vi "BT_pass_fail.vi"(8 "error in":errorcluster, 9 "BT Item result Input":dbl, 10 "BT Item Name Input":string="ACP_MAX_POWER_DBM_OFFSET_-5:", 11 "BT Test Text Input":string="TX_BDR 2402 DH1") -> (0 "error out":errorcluster, 2 "Pass?(string)":string, 3 "Pass?(boolen)":bool)   [LabVIEW 2012]
uses:
  <vilib>/Utility/file.llb/Read From Spreadsheet File (string).vi
panel:
  out "High limit":dbl
  out "Lower limit":dbl
  out "BT_RX_EDR":string[][](array[string])
  out "output 3":string
  out "Frequency":dbl
  out "BT test item":string
  in  "BT_Range":T1={"BT_TX_BDR"=[["POWER_AVERAGE_DBM", "-6", "4", "", "", "", "", "", "", "", "", "", "", "", ""], ["POWER_PEAK_DBM", "", "23", "", "", "", "", "", "", "", "", "", "", "", ""], ["DELTA_F2_MAX_ACCESS", "115", "", "", "", "", "", "", "", "", "", "", "", "", ""], ["ACP_MAX_POWER_DBM_OFFSET_-5", "", "-40", "", "", "", "", "", "", "", "", "", "", "", ""], ["ACP_MAX_POWER_DBM_OFFSET_-4", "", "-40", "", "", "", "", "", "", "", "", "", "", "", ""], ["ACP_MAX_POWER_DBM_OFFSET_-3", "", "-40", "", "", "", "", "", "", "", "", "", "", "", ""], ["ACP_MAX_POWER_DBM_OFFSET_-2", "", "-40", "", "", "", "", "", "", "", "", "", "", "", ""], ["ACP_MAX_POWER_DBM_OFFSET_-1", "", "-20", "", "", "", "", "", "", "", "", "", "", "", ""], ["ACP_MAX_POWER_DBM_OFFSET_1", "", "-20", "", "", "", "", "", "", "", "", "", "", "", ""], ["ACP_MAX_POWER_DBM_OFFSET_2", "", "-40", "", "", "", "", "", "", "", "", "", "", "", ""], ["ACP_MAX_POWER_DBM_OFFSET_3", "", "-40", "", "", "", "", "", "", "", "", "", "", "", ""], ["ACP_MAX_POWER_DBM_OFFSET_4", "", "-40", "", "", "", "", "", "", "", "", "", "", "", ""], ["ACP_MAX_POWER_DBM_OFFSET_5", "", "-40", "", "", "", "", "", "", "", "", "", "", "", ""]], "BT_TX_EDR"=[["EDR_OMEGA_I", "-75", "75", "", "", "", "", "", "", "", "", "", "", "", ""], ["EDR_POW_DIFF_DB", "-4", "1", "", "", "", "", "", "", "", "", "", "", "", ""], ["EDR_EVM_AV", "", "13", "", "", "", "", "", "", "", "", "", "", "", ""], ["EDR_EVM_PK", "", "25", "", "", "", "", "", "", "", "", "", "", "", ""], ["EDR_PROB_EVM_99_PASS", "100", "100", "", "", "", "", "", "", "", "", "", "", "", ""], ["POWER_AVERAGE_DBM", "-6", "4", "", "", "", "", "", "", "", "", "", "", "", ""], ["ACP_MAX_POWER_DBM_OFFSET_-5", "", "-40", "", "", "", "", "", "", "", "", "", "", "", ""], ["ACP_MAX_POWER_DBM_OFFSET_-4", "", "-40", "", "", "", "", "", "", "", "", "", "", "", ""], ["ACP_MAX_POWER_DBM_OFFSET_-3", "", "-40", "", "", "", "", "", "", "", "", "", "", "", ""], ["ACP_MAX_POWER_DBM_OFFSET_-2", "", "-20", "", "", "", "", "", "", "", "", "", "", "", ""], ["ACP_MAX_POWER_DB_OFFSET_-1", "", "-26", "", "", "", "", "", "", "", "", "", "", "", ""], ["ACP_MAX_POWER_DB_OFFSET_1", "", "-26", "", "", "", "", "", "", "", "", "", "", "", ""], ["ACP_MAX_POWER_DBM_OFFSET_2", "", "-20", "", "", "", "", "", "", "", "", "", "", "", ""], ["ACP_MAX_POWER_DBM_OFFSET_3", "", "-40", "", "", "", "", "", "", "", "", "", "", "", ""], ["ACP_MAX_POWER_DBM_OFFSET_4", "", "-40", "", "", "", "", "", "", "", "", "", "", "", ""], ["ACP_MAX_POWER_DBM_OFFSET_5", "", "-40", "", "", "", "", "", "", "", "", "", "", "", ""]], "BT_RX_BDR"=[["BER", "", "0.1", "", "", "", "", "", "", "", "", "", "", "", ""]], "BT_RX_EDR"=[["BER", "", "0.1", "", "", "", "", "", "", "", "", "", "", "", ""]]}
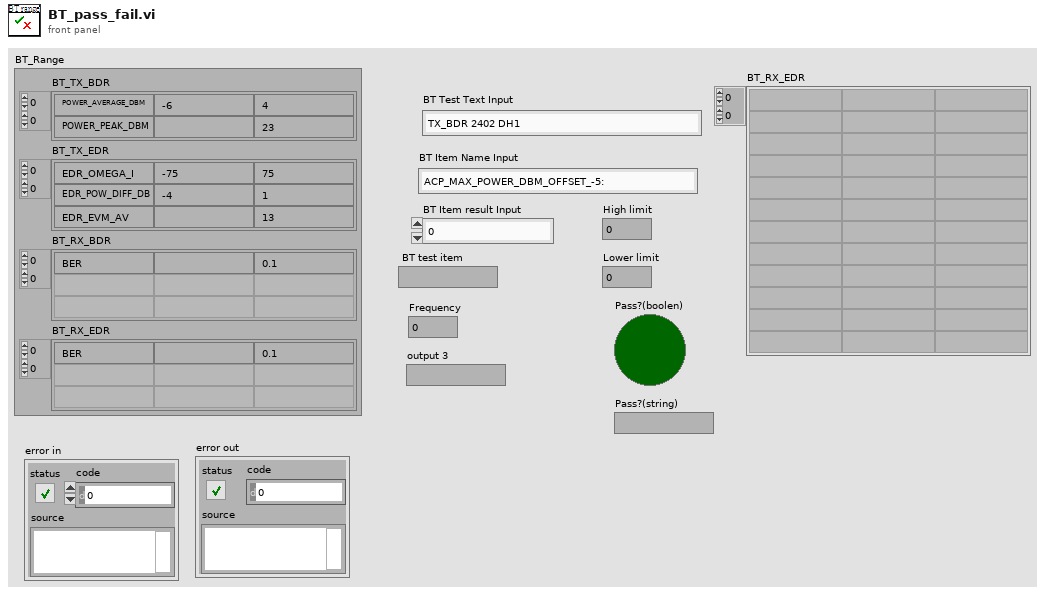
[diagram p1: front panel]
types:
  T1 = cluster{"BT_TX_BDR":string[][], "BT_TX_EDR":string[][], "BT_RX_BDR":string[][], "BT_RX_EDR":string[][]}
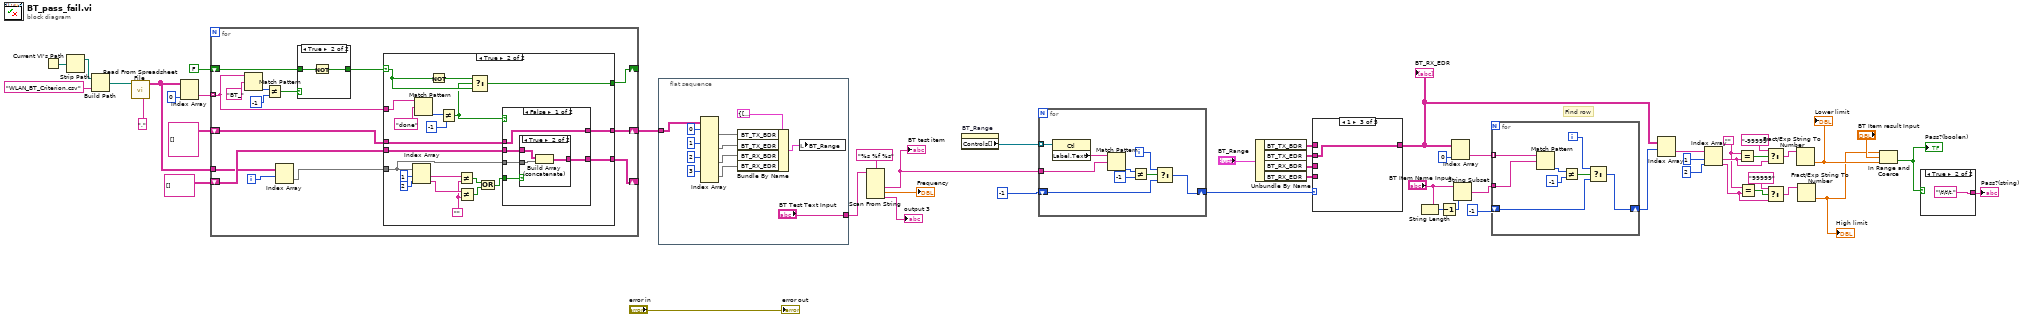
[diagram p0: block diagram]
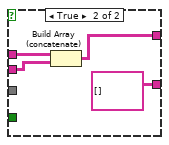
[diagram p4: hidden frame]
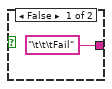
[diagram p6: hidden frame]
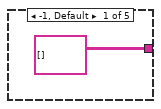
[diagram p7: hidden frame]
diagram:
  w23 = ""
  # "Find row"
  n1 = Current VI's Path() -> (path=w13:path)
  n2 = Strip Path(path=w13) -> (stripped path=w12:path)  [unwired: 1 out]
  n3 = Build Path(base path=w12, name or relative path="WLAN_BT_Criterion.csv") -> (appended path=w10:path)
  n4 = call-poly <vilib>:"Read From Spreadsheet File.vi"("delimiter (\\t)"="," ("delimiter (\\t)"), "file path (dialog if empty)"=w10) -> ("all rows"=w4:string[][])  [unwired: 5 in, 4 out]
  n5 = Index Array(array=w4, index (col)=0 ("disabled index (col)")) -> (element=w5:string[])  [unwired: 1 in]
  n6 = for {
    tunnel: w5 -> [w56] mode=indexing
    shift-right: [w55] -> _
    shift-left: FALSE ("Strat to store date") -> [w63]
    shift-right: [w60] -> _
    shift-left: string[][] [] -> [w61]
    tunnel: w4 -> [w59]
    shift-right: [w53] -> w1
    shift-left: string[][][] [] -> [w54]
    i -> [w58]
    n7 = Match Pattern(string=w56, regular expression="BT_") -> (offset past match=w66:i32)  [unwired: 1 in, 3 out]
    n8 = Not Equal?(x=w66, y=-1) -> (x != y?=w64:bool)
    n9 = Index Array(array=w59, index (row)=w58) -> (element=w57:string[])  [unwired: 1 in]
    n10 = case shown="True" w64 {
      tunnel: [w105 w106] -> w62
      tunnel: w63 -> [w105 w107]
      frame False {
      }
      frame True {
        n11 = Not(x=w107) -> (.not. x?=w106:bool)
      }
    }
    n12 = case shown="True" w62 {
      selector: w62 -> [w69 w78]
      tunnel: w61 -> [w70 w84]
      tunnel: w57 -> [_ w74]
      tunnel: [w70 w83] -> w60
      tunnel: w56 -> [_ w81]
      tunnel: [w69 w76] -> w55
      tunnel: w54 -> [w68 w72]
      tunnel: [w68 w71] -> w53
      frame False {
      }
      frame True {
        w87 = ""
        n13 = Index Array(array=w74, index #1=1 ("index"), index #2=2 ("index")) -> (element #1=w89:string, element #2=w88:string)
        n14 = Match Pattern(string=w81, regular expression="done") -> (offset past match=w80:i32)  [unwired: 1 in, 3 out]
        n15 = Not(x=w78) -> (.not. x?=w77:bool)
        n16 = Not Equal?(x=w80, y=-1) -> (x != y?=w73:bool)
        n17 = Not Equal?(x=w89, y=w87) -> (x != y?=w86:bool)
        n18 = Not Equal?(x=w88, y=w87) -> (x != y?=w85:bool)
        n19 = Select(t=w77, s=w73, f=w78) -> (s? t:f=w76:bool)
        n20 = Or(x=w86, y=w85) -> (x .or. y?=w75:bool)
        n21 = case shown="False" w73 {
          tunnel: w84 -> [w96 w102]
          tunnel: [w95 string[][] []] -> w83
          tunnel: w75 -> [w94 _]
          tunnel: w74 -> [w93 _]
          tunnel: w72 -> [w92 w103]
          tunnel: [w92 w101] -> w71
          frame False {
            n22 = case shown="True" w94 {
              tunnel: w96 -> [w97 w100]
              tunnel: [w97 w99] -> w95
              tunnel: w93 -> [_ w98]
              frame False {
              }
              frame True {
                n23 = Build Array (concatenate)(w100, w98) -> (w99:string[][])
              }
            }
          }
          frame True {
            n24 = Build Array (concatenate)(w103, w102) -> (w101:string[][][])
          }
        }
      }
    }
  }
  n25 = flat-sequence {
    tunnel: ["BT Test Text Input"] -> w52
    tunnel: w1 -> [w118]
    frame #0 {
      n26 = Index Array(array=w118, index (dim 0) #1=0 ("index (page)"), index (dim 0) #2=1 ("index (page)"), index (dim 0) #3=2 ("index (page)"), index (dim 0) #4=3 ("index (page)")) -> (element #1=w111:string[][], element #2=w110:string[][], element #3=w109:string[][], element #4=w108:string[][])  [unwired: 8 in]
      n27 = Bundle By Name(cluster=T1 {"BT_TX_BDR"=[["POWER_AVERAGE_DBM", "-6", "4", "", "", "", "", "", "", "", "", "", "", "", ""], ["POWER_PEAK_DBM", "", "23", "", "", "", "", "", "", "", "", "", "", "", ""], ["DELTA_F2_MAX_ACCESS", "115", "", "", "", "", "", "", "", "", "", "", "", "", ""], ["ACP_MAX_POWER_DBM_OFFSET_-5", "", "-40", "", "", "", "", "", "", "", "", "", "", "", ""], ["ACP_MAX_POWER_DBM_OFFSET_-4", "", "-40", "", "", "", "", "", "", "", "", "", "", "", ""], ["ACP_MAX_POWER_DBM_OFFSET_-3", "", "-40", "", "", "", "", "", "", "", "", "", "", "", ""], ["ACP_MAX_POWER_DBM_OFFSET_-2", "", "-40", "", "", "", "", "", "", "", "", "", "", "", ""], ["ACP_MAX_POWER_DBM_OFFSET_-1", "", "-20", "", "", "", "", "", "", "", "", "", "", "", ""], ["ACP_MAX_POWER_DBM_OFFSET_1", "", "-20", "", "", "", "", "", "", "", "", "", "", "", ""], ["ACP_MAX_POWER_DBM_OFFSET_2", "", "-40", "", "", "", "", "", "", "", "", "", "", "", ""], ["ACP_MAX_POWER_DBM_OFFSET_3", "", "-40", "", "", "", "", "", "", "", "", "", "", "", ""], ["ACP_MAX_POWER_DBM_OFFSET_4", "", "-40", "", "", "", "", "", "", "", "", "", "", "", ""], ["ACP_MAX_POWER_DBM_OFFSET_5", "", "-40", "", "", "", "", "", "", "", "", "", "", "", ""]], "BT_TX_EDR"=[["EDR_OMEGA_I", "-75", "75", "", "", "", "", "", "", "", "", "", "", "", ""], ["EDR_POW_DIFF_DB", "-4", "1", "", "", "", "", "", "", "", "", "", "", "", ""], ["EDR_EVM_AV", "", "13", "", "", "", "", "", "", "", "", "", "", "", ""], ["EDR_EVM_PK", "", "25", "", "", "", "", "", "", "", "", "", "", "", ""], ["EDR_PROB_EVM_99_PASS", "100", "100", "", "", "", "", "", "", "", "", "", "", "", ""], ["POWER_AVERAGE_DBM", "-6", "4", "", "", "", "", "", "", "", "", "", "", "", ""], ["ACP_MAX_POWER_DBM_OFFSET_-5", "", "-40", "", "", "", "", "", "", "", "", "", "", "", ""], ["ACP_MAX_POWER_DBM_OFFSET_-4", "", "-40", "", "", "", "", "", "", "", "", "", "", "", ""], ["ACP_MAX_POWER_DBM_OFFSET_-3", "", "-40", "", "", "", "", "", "", "", "", "", "", "", ""], ["ACP_MAX_POWER_DBM_OFFSET_-2", "", "-20", "", "", "", "", "", "", "", "", "", "", "", ""], ["ACP_MAX_POWER_DB_OFFSET_-1", "", "-26", "", "", "", "", "", "", "", "", "", "", "", ""], ["ACP_MAX_POWER_DB_OFFSET_1", "", "-26", "", "", "", "", "", "", "", "", "", "", "", ""], ["ACP_MAX_POWER_DBM_OFFSET_2", "", "-20", "", "", "", "", "", "", "", "", "", "", "", ""], ["ACP_MAX_POWER_DBM_OFFSET_3", "", "-40", "", "", "", "", "", "", "", "", "", "", "", ""], ["ACP_MAX_POWER_DBM_OFFSET_4", "", "-40", "", "", "", "", "", "", "", "", "", "", "", ""], ["ACP_MAX_POWER_DBM_OFFSET_5", "", "-40", "", "", "", "", "", "", "", "", "", "", "", ""]], "BT_RX_BDR"=[["BER", "", "0.1", "", "", "", "", "", "", "", "", "", "", "", ""]], "BT_RX_EDR"=[["BER", "", "0.1", "", "", "", "", "", "", "", "", "", "", "", ""]]} ("BT_Range"), "BT_TX_BDR"=w111, "BT_TX_EDR"=w110, "BT_RX_BDR"=w109, "BT_RX_EDR"=w108) -> (w112:T1)
      n28 = local write "BT_Range"(w112) -> ()
    }
  }
  n29 = Scan From String(format string="%s %f %s", input string=w52) -> (output 1=w46:string, output 2=→"Frequency":dbl, output 3=→"output 3":string)  [unwired: 5 in, 3 out]
  "BT test item" <- w46
  n30 = property on="BT_Range" class="Clust (strict)"() -> ("Controls[]"=w48:refnum<vi>[])  [unwired: 2 in, 2 out]
  n31 = for {
    tunnel: w48 -> [w128] mode=indexing
    tunnel: w46 -> [w126]
    shift-right: [w120] -> w44
    shift-left: -1 -> [w121]
    i -> [w122]
    n32 = property class="Ctl"(reference=w128) -> ("Label.Text"=w127:string)  [unwired: 1 in, 2 out]
    n33 = Match Pattern(string=w127, regular expression=w126) -> (offset past match=w125:i32)  [unwired: 1 in, 3 out]
    n34 = Not Equal?(x=w125, y=-1) -> (x != y?=w123:bool)
    n35 = Select(t=w122, s=w123, f=w121) -> (s? t:f=w120:i32)
  }
  n36 = Unbundle By Name("BT_Range") -> ("BT_TX_BDR"=w43:string[][], "BT_TX_EDR"=w42:string[][], "BT_RX_BDR"=w41:string[][], "BT_RX_EDR"=w40:string[][])
  n37 = case shown="1" w44 {
    tunnel: w43 -> [_ w130 _ _ _]
    tunnel: w42 -> [_ _ w131 _ _]
    tunnel: w41 -> [_ _ _ w132 _]
    tunnel: w40 -> [_ _ _ _ w133]
    tunnel: [string[][] [] ("BT_RX_EDR") w130 w131 w132 w133] -> w32
    frame -1, Default {
    }
    frame 0 {
    }
    frame 1 {
    }
    frame 2 {
    }
    frame 3 {
    }
  }
  "BT_RX_EDR" <- w32
  n38 = String Length(string="BT Item Name Input") -> (length=w35:i32)
  n39 = Decrement(x=w35) -> (x-1=w34:i32)
  n40 = Index Array(array=w32, index (col)=0 ("disabled index (col)")) -> (element=w38:string[])  [unwired: 1 in]
  n41 = String Subset(string="BT Item Name Input", length (rest)=w34) -> (substring=w33:string)  [unwired: 1 in]
  n42 = for {
    tunnel: w38 -> [w141] mode=indexing
    tunnel: w33 -> [w140]
    shift-right: [w134] -> w31
    shift-left: -1 -> [w135]
    i -> [w136]
    n43 = Match Pattern(string=w141, regular expression=w140) -> (offset past match=w139:i32)  [unwired: 1 in, 3 out]
    n44 = Not Equal?(x=w139, y=-1) -> (x != y?=w137:bool)
    n45 = Select(t=w136, s=w137, f=w135) -> (s? t:f=w134:i32)
  }
  n46 = Index Array(array=w32, index (row)=w31) -> (element=w30:string[])  [unwired: 1 in]
  n47 = Index Array(array=w30, index #1=1 ("index"), index #2=2 ("index")) -> (element #1=w26:string, element #2=w22:string)
  n48 = Equal?(x=w23, y=w26) -> (x = y?=w27:bool)
  n49 = Equal?(x=w23, y=w22) -> (x = y?=w24:bool)
  n50 = Select(t="-99999", s=w27, f=w26) -> (s? t:f=w20:string)
  n51 = Select(t="99999", s=w24, f=w22) -> (s? t:f=w19:string)
  n52 = Fract/Exp String To Number(string=w20) -> (number=w17:dbl)  [unwired: 3 in, 1 out]
  "Lower limit" <- w17
  n53 = Fract/Exp String To Number(string=w19) -> (number=w16:dbl)  [unwired: 3 in, 1 out]
  "High limit" <- w16
  n54 = In Range and Coerce(upper limit=w16, x="BT Item result Input", lower limit=w17) -> (In Range?=w15:bool)  [unwired: 1 out]
  "Pass?(boolen)" <- w15
  n55 = case shown="True" w15 {
    tunnel: ["\t\t\tFail" "\t\t\t."] -> w14
    frame False {
    }
    frame True {
    }
  }
  "Pass?(string)" <- w14
  "error out" <- "error in"
